vi "Begin.vi"(8 "error in":errorcluster) -> (0 "error out":errorcluster)   [LabVIEW 2019]
doc: "Called before other user functions, this VI can be used to open I/O refnums, load in file data, and do general program initialization. Notice that the <B>error out</B> terminal is simply used for data flow. Wiring it to other structures or subVIs ensures that this VI runs first."
uses:
  Robot Global Data.vi
  <vilib>/Rock Robotics/WPI/DriverStation/WPI_DriverStationRobotMode2.ctl
  <vilib>/Rock Robotics/WPI/Joystick/WPI_JoystickDeviceEnum.ctl
  <vilib>/Rock Robotics/Network Tables/NT Write String Array.vi
  <vilib>/Rock Robotics/WPI/RobotDrive/WPI_RobotDriveOpen2MotorWithExistingMotors.vi
  <vilib>/Rock Robotics/WPI/MotorControl/WPI_MotorControlOpen SPARK.vi
  <vilib>/Rock Robotics/SystemInterfaces/DIO/FPGA_DIOPWMChannel.ctl
  <vilib>/Rock Robotics/WPI/SafetyOutput/WPI_SafetyOutputConfigMenu.ctl
  <vilib>/Rock Robotics/Network Tables/NT Write Numeric Array.vi
  <vilib>/Rock Robotics/Network Tables/NT Write Boolean Array.vi
  <vilib>/Rock Robotics/WPI/Solenoid/WPI_SolenoidOpenSingle.vi
  <vilib>/Rock Robotics/WPI/Solenoid/WPI_SolenoidSetEnum.vi
  <vilib>/Rock Robotics/WPI/Solenoid/WPI_SolenoidChannel.ctl
  <vilib>/Rock Robotics/WPI/Solenoid/WPI_SolenoidValue.ctl
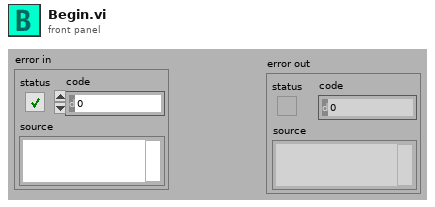
[diagram p1: front panel]
types:
  T1 = typedef "WPI_JoystickDeviceEnum.ctl" = enum16{"USB 0", "USB 1", "USB 2", "USB 3", "USB 4", "USB 5"}
  T2 = typedef "WPI_DriverStationRobotMode2.ctl" = enum16{"Autonomous Disabled", "Autonomous Enabled", "Teleop Disabled", "Teleop Enabled", "Disconnected", "Finish", "Test Disabled", "Test Enabled", "Emergency Stopped"}
  T3 = typedef "WPI_JoystickDevRef.ctl" = cluster{"Device":T1}
  T4 = typedef "WPI_MotorControlDeviceRef.ctl" = cluster{"DeviceStatus":errorcluster, "Type":T5, "PWM":cluster{"PWM Channel":T6, "DeadBand":T7}, "CAN":cluster{"Device Number":u8, "SetOutput VI Ref":variant, "GetOutput VI Ref":variant, "Enable VI Ref":variant, "Disable VI Ref":variant, "Data":variant}, "Invert":bool, "DIO PWM":cluster{"PWM \"Enable\" Channel":T6, "DIOChannel":T8, "PWM Rate":dbl}}
  T5 = typedef "WPI_MotorControlType.ctl" = enum16{"PWM", "CAN", "DIO PWM"}
  T6 = typedef "FPGA_DIOPWMChannel.ctl" = enum8{"PWM 0", "PWM 1", "PWM 2", "PWM 3", "PWM 4", "PWM 5", "PWM 6", "PWM 7", "PWM 8", "PWM 9", "PWM MXP 0", "PWM MXP 1", "PWM MXP 2", "PWM MXP 3", "PWM MXP 4", "PWM MXP 5", "PWM MXP 6", "PWM MXP 7", "PWM MXP 8", "PWM MXP 9", "Invalid"}
  T7 = typedef "WPI_PWMDeadband.ctl" = cluster{"Name":string, "maxPositivePwm":i32, "minPositivePwm":i32, "centerPwm":i32, "maxNegativePwm":i32, "minNegativePwm":i32, "angularRange":u16}
  T8 = typedef "FPGA_DIOChannel.ctl" = enum8{"DIO 0", "DIO 1", "DIO 2", "DIO 3", "DIO 4", "DIO 5", "DIO 6", "DIO 7", "DIO 8", "DIO 9", "DIO MXP 0", "DIO MXP 1", "DIO MXP 2", "DIO MXP 3", "DIO MXP 4", "DIO MXP 5", "DIO MXP 6", "DIO MXP 7", "DIO MXP 8", "DIO MXP 9", "DIO MXP 10", "DIO MXP 11", "DIO MXP 12", "DIO MXP 13", "DIO MXP 14", "DIO MXP 15", "SPI Port CS1", "SPI Port CS2", "SPI Port CS3", "SPI Port MISO", "SPI Port MOSI", "Invalid"}
  T9 = typedef "WPI_SafetyOutputConfigMenu.ctl" = enum16{"Enable", "Disable"}
  T10 = typedef "WPI_RobotDriveDevRef.ctl" = cluster{"DevStatus":errorcluster, "Motors[]":T4[], "Square Inputs":bool, "Max Output":dbl}
  T11 = typedef "WPI_SolenoidValue.ctl" = enum16{"Off", "On", "Forward", "Reverse"}
  T12 = typedef "WPI_SolenoidChannel.ctl" = enum8{"Solenoid 0", "Solenoid 1", "Solenoid 2", "Solenoid 3", "Solenoid 4", "Solenoid 5", "Solenoid 6", "Solenoid 7", "Invalid"}
  T13 = typedef "WPI_SolenoidDevRef.ctl" = cluster{"DevStatus":errorcluster, "Pneumatics Control Module":u8, "Forward Solenoid Channel":T12, "Reverse Solenoid Channel":T12}
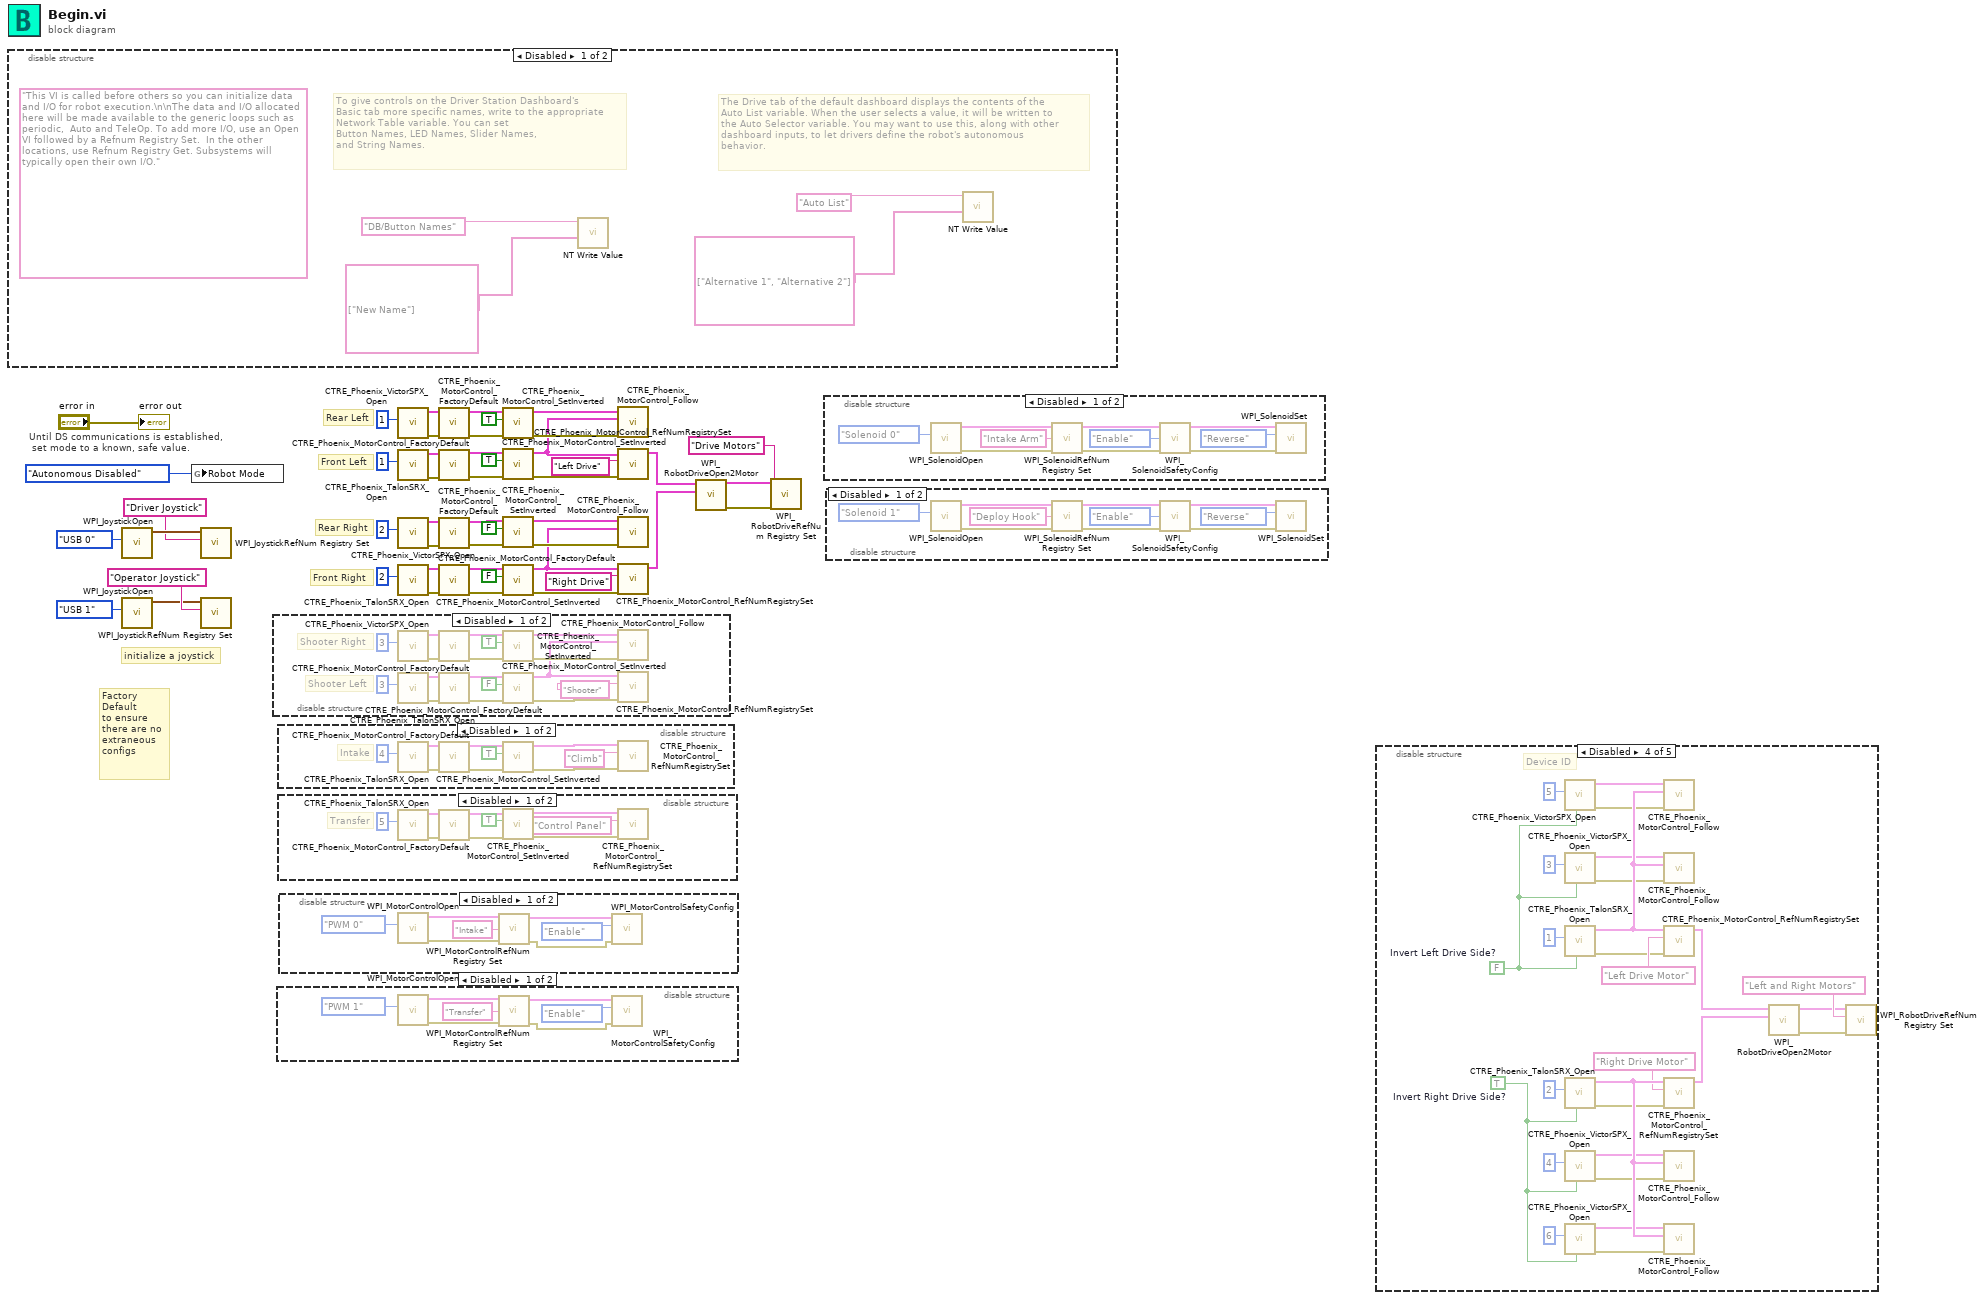
[diagram p0: block diagram]
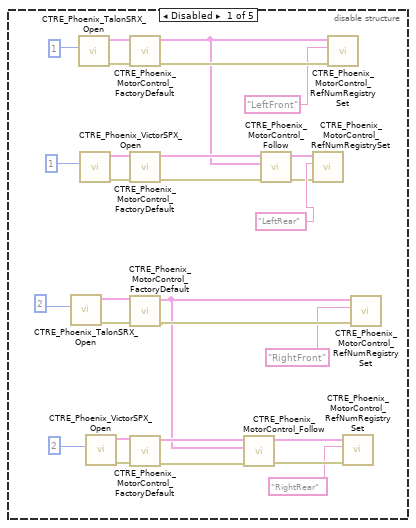
[diagram p9: hidden frame]
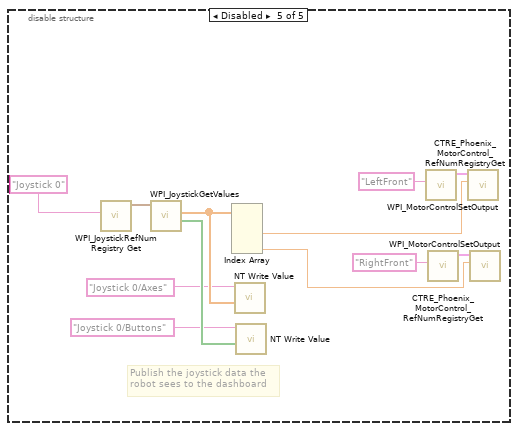
[diagram p12: hidden frame]
diagram:
  # "Factory \nDefault \nto ensure \nthere are no \nextraneous \nconfigs"
  # "Front Right"
  # "Front Left"
  # "Rear Right"
  # "Rear Left"
  # "initialize a joystick"
  # "Until DS communications is established,\n set mode to a known, safe value."
  n1 = disable-structure shown="Disabled" {
    frame Disabled {
      (unwired) "This VI is called before others so you can initialize data and I/O for robot execution.\n\nThe data and I/O allocated here will be made available to the generic loops such as periodic,  Auto and TeleOp. To add more I/O, use an Open VI followed by a Refnum Registry Set.  In the other locations, use Refnum Registry Get. Subsystems will typically open their own I/O."
      # "The Drive tab of the default dashboard displays the contents of the\nAuto List variable. When the user selects a value, it will be written to\nthe Auto Selector variable. You may want to use this, along with other\ndashboard inputs, to let drivers define the robot's autonomous\nbehavior."
      # "To give controls on the Driver Station Dashboard's\nBasic tab more specific names, write to the appropriate\nNetwork Table variable. You can set\nButton Names, LED Names, Slider Names,\nand String Names."
      n2 = call-poly <vilib>:"NT Write Value.vi"("String Array"=string[] ["New Name"], "Name"="DB/Button Names") -> ()  [unwired: 9 in, 1 out]
      n3 = call-poly <vilib>:"NT Write Value.vi"("String Array"=string[] ["Alternative 1", "Alternative 2"], "Name"="Auto List") -> ()  [unwired: 9 in, 1 out]
    }
    frame Enabled {
    }
  }
  n4 = call <vilib>:"WPI_JoystickOpen.vi"("JoystickDevice"=WPI_JoystickDeviceEnum."USB 0") -> ("JoystickDevRef"=w30:T3)  [unwired: 10 in]
  n5 = call <vilib>:"WPI_JoystickOpen.vi"("JoystickDevice"=WPI_JoystickDeviceEnum."USB 1") -> ("JoystickDevRef"=w45:T3)  [unwired: 10 in]
  n6 = global write "Robot Global Data.vi" "Robot Mode"(WPI_DriverStationRobotMode2."Autonomous Disabled" ("Robot Mode")) -> ()
  n7 = call <vilib>:"WPI_JoystickRefNum Registry Set.vi"("refnum name"="Driver Joystick", "JoystickDevRef"=w30) -> ()  [unwired: 8 in, 2 out]
  n8 = call <vilib>:"WPI_JoystickRefNum Registry Set.vi"("refnum name"="Operator Joystick", "JoystickDevRef"=w45) -> ()  [unwired: 8 in, 2 out]
  n9 = disable-structure shown="Disabled" {
    frame Disabled {
      # "Shooter Left"
      # "Shooter Right"
      n10 = call <vilib>:"CTRE_Phoenix_VictorSPX_Open.vi"("Device Number"=u8 3) -> ("error out"=w65:errorcluster, "CAN Talon SRX Ref"=w64:T4)  [unwired: 9 in]
      n11 = call <vilib>:"CTRE_Phoenix_TalonSRX_Open.vi"("Device Number"=u8 3) -> ("error out"=w63:errorcluster, "CAN Talon SRX Ref"=w62:T4)  [unwired: 9 in]
      n12 = call <vilib>:"CTRE_Phoenix_MotorControl_FactoryDefault.vi"("error in"=w65, "PhoenixMotorControlDevRef"=w64) -> ("error out"=w59:errorcluster, "PhoenixMotorControlDevRef"=w60:T4)  [unwired: 8 in]
      n13 = call <vilib>:"CTRE_Phoenix_MotorControl_FactoryDefault.vi"("error in"=w63, "PhoenixMotorControlDevRef"=w62) -> ("error out"=w54:errorcluster, "PhoenixMotorControlDevRef"=w55:T4)  [unwired: 8 in]
      n14 = call <vilib>:"CTRE_Phoenix_MotorControl_SetInverted.vi"("error in (no error)"=w59, "Invert?"=TRUE, "PhoenixMotorControlDevRef"=w60) -> ("error out"=w58:errorcluster, "PhoenixMotorControlDevRef"=w57:T4)  [unwired: 7 in]
      n15 = call <vilib>:"CTRE_Phoenix_MotorControl_SetInverted.vi"("error in (no error)"=w54, "Invert?"=FALSE, "PhoenixMotorControlDevRef"=w55) -> ("error out"=w53:errorcluster, "PhoenixMotorControlDevRef"=w52:T4)  [unwired: 7 in]
      n16 = call <vilib>:"CTRE_Phoenix_MotorControl_Follow.vi"("error in (no error)"=w58, "Master Controller to Follow"=w52, "PhoenixMotorControlDevRef"=w57) -> ()  [unwired: 7 in, 2 out]
      n17 = call <vilib>:"CTRE_Phoenix_MotorControl_RefNumRegistrySet.vi"("error in (no error)"=w53, "refnum name"="Shooter", "PhoenixMotorControlDevRef"=w52) -> ()  [unwired: 7 in, 2 out]
    }
    frame Enabled {
    }
  }
  n18 = disable-structure shown="Disabled" {
    frame Disabled {
      n19 = call-poly <vilib>:"WPI_MotorControlOpen.vi"("PWM Channel"=FPGA_DIOPWMChannel."PWM 1") -> ("error out"=w74:errorcluster, "MotorControlDeviceRef"=w70:T4)  [unwired: 9 in]
      n20 = call <vilib>:"WPI_MotorControlRefNum Registry Set.vi"("error in (no error)"=w74, "refnum name"="Transfer", "MotorControlDevRef"=w70) -> ("error out"=w75:errorcluster, "MotorControlDevRef"=w71:T4)  [unwired: 7 in]
      n21 = call <vilib>:"WPI_MotorControlSafetyConfig.vi"("error in (no error)"=w75, "mode"=WPI_SafetyOutputConfigMenu."Enable", "MotorControlDevRef"=w71) -> ()  [unwired: 7 in, 2 out]
    }
    frame Enabled {
    }
  }
  n22 = disable-structure shown="Disabled" {
    frame Disabled {
      # "Intake"
      n23 = call <vilib>:"CTRE_Phoenix_TalonSRX_Open.vi"("Device Number"=u8 4) -> ("error out"=w82:errorcluster, "CAN Talon SRX Ref"=w81:T4)  [unwired: 9 in]
      n24 = call <vilib>:"CTRE_Phoenix_MotorControl_FactoryDefault.vi"("error in"=w82, "PhoenixMotorControlDevRef"=w81) -> ("error out"=w78:errorcluster, "PhoenixMotorControlDevRef"=w79:T4)  [unwired: 8 in]
      n25 = call <vilib>:"CTRE_Phoenix_MotorControl_SetInverted.vi"("error in (no error)"=w78, "Invert?"=TRUE, "PhoenixMotorControlDevRef"=w79) -> ("error out"=w77:errorcluster, "PhoenixMotorControlDevRef"=w76:T4)  [unwired: 7 in]
      n26 = call <vilib>:"CTRE_Phoenix_MotorControl_RefNumRegistrySet.vi"("error in (no error)"=w77, "refnum name"="Climb", "PhoenixMotorControlDevRef"=w76) -> ()  [unwired: 7 in, 2 out]
    }
    frame Enabled {
    }
  }
  n27 = disable-structure shown="Disabled" {
    frame Disabled {
      # "Transfer"
      n28 = call <vilib>:"CTRE_Phoenix_TalonSRX_Open.vi"("Device Number"=u8 5) -> ("error out"=w91:errorcluster, "CAN Talon SRX Ref"=w90:T4)  [unwired: 9 in]
      n29 = call <vilib>:"CTRE_Phoenix_MotorControl_FactoryDefault.vi"("error in"=w91, "PhoenixMotorControlDevRef"=w90) -> ("error out"=w87:errorcluster, "PhoenixMotorControlDevRef"=w88:T4)  [unwired: 8 in]
      n30 = call <vilib>:"CTRE_Phoenix_MotorControl_SetInverted.vi"("error in (no error)"=w87, "Invert?"=TRUE, "PhoenixMotorControlDevRef"=w88) -> ("error out"=w86:errorcluster, "PhoenixMotorControlDevRef"=w85:T4)  [unwired: 7 in]
      n31 = call <vilib>:"CTRE_Phoenix_MotorControl_RefNumRegistrySet.vi"("error in (no error)"=w86, "refnum name"="Control Panel", "PhoenixMotorControlDevRef"=w85) -> ()  [unwired: 7 in, 2 out]
    }
    frame Enabled {
    }
  }
  n32 = disable-structure shown="Disabled" {
    frame Disabled {
      n33 = call-poly <vilib>:"WPI_MotorControlOpen.vi"("PWM Channel"=FPGA_DIOPWMChannel."PWM 0") -> ("error out"=w95:errorcluster, "MotorControlDeviceRef"=w99:T4)  [unwired: 9 in]
      n34 = call <vilib>:"WPI_MotorControlRefNum Registry Set.vi"("error in (no error)"=w95, "refnum name"="Intake", "MotorControlDevRef"=w99) -> ("error out"=w94:errorcluster, "MotorControlDevRef"=w98:T4)  [unwired: 7 in]
      n35 = call <vilib>:"WPI_MotorControlSafetyConfig.vi"("error in (no error)"=w94, "mode"=WPI_SafetyOutputConfigMenu."Enable", "MotorControlDevRef"=w98) -> ()  [unwired: 7 in, 2 out]
    }
    frame Enabled {
    }
  }
  n36 = call <vilib>:"CTRE_Phoenix_VictorSPX_Open.vi"("Device Number"=u8 1) -> ("error out"=w28:errorcluster, "CAN Talon SRX Ref"=w27:T4)  [unwired: 9 in]
  n37 = call <vilib>:"CTRE_Phoenix_TalonSRX_Open.vi"("Device Number"=u8 1) -> ("error out"=w25:errorcluster, "CAN Talon SRX Ref"=w26:T4)  [unwired: 9 in]
  n38 = call <vilib>:"CTRE_Phoenix_VictorSPX_Open.vi"("Device Number"=u8 2) -> ("error out"=w24:errorcluster, "CAN Talon SRX Ref"=w23:T4)  [unwired: 9 in]
  n39 = call <vilib>:"CTRE_Phoenix_TalonSRX_Open.vi"("Device Number"=u8 2) -> ("error out"=w22:errorcluster, "CAN Talon SRX Ref"=w21:T4)  [unwired: 9 in]
  n40 = call <vilib>:"CTRE_Phoenix_MotorControl_FactoryDefault.vi"("error in"=w28, "PhoenixMotorControlDevRef"=w27) -> ("error out"=w19:errorcluster, "PhoenixMotorControlDevRef"=w18:T4)  [unwired: 8 in]
  n41 = call <vilib>:"CTRE_Phoenix_MotorControl_FactoryDefault.vi"("error in"=w25, "PhoenixMotorControlDevRef"=w26) -> ("error out"=w13:errorcluster, "PhoenixMotorControlDevRef"=w14:T4)  [unwired: 8 in]
  n42 = call <vilib>:"CTRE_Phoenix_MotorControl_FactoryDefault.vi"("error in"=w24, "PhoenixMotorControlDevRef"=w23) -> ("error out"=w9:errorcluster, "PhoenixMotorControlDevRef"=w8:T4)  [unwired: 8 in]
  n43 = call <vilib>:"CTRE_Phoenix_MotorControl_FactoryDefault.vi"("error in"=w22, "PhoenixMotorControlDevRef"=w21) -> ("error out"=w4:errorcluster, "PhoenixMotorControlDevRef"=w3:T4)  [unwired: 8 in]
  n44 = call <vilib>:"CTRE_Phoenix_MotorControl_SetInverted.vi"("error in (no error)"=w19, "Invert?"=TRUE, "PhoenixMotorControlDevRef"=w18) -> ("error out"=w16:errorcluster, "PhoenixMotorControlDevRef"=w17:T4)  [unwired: 7 in]
  n45 = call <vilib>:"CTRE_Phoenix_MotorControl_SetInverted.vi"("error in (no error)"=w13, "Invert?"=TRUE, "PhoenixMotorControlDevRef"=w14) -> ("error out"=w12:errorcluster, "PhoenixMotorControlDevRef"=w11:T4)  [unwired: 7 in]
  n46 = call <vilib>:"CTRE_Phoenix_MotorControl_SetInverted.vi"("error in (no error)"=w9, "Invert?"=FALSE, "PhoenixMotorControlDevRef"=w8) -> ("error out"=w6:errorcluster, "PhoenixMotorControlDevRef"=w7:T4)  [unwired: 7 in]
  n47 = call <vilib>:"CTRE_Phoenix_MotorControl_SetInverted.vi"("error in (no error)"=w4, "Invert?"=FALSE, "PhoenixMotorControlDevRef"=w3) -> ("error out"=w1:errorcluster, "PhoenixMotorControlDevRef"=w2:T4)  [unwired: 7 in]
  n48 = call <vilib>:"CTRE_Phoenix_MotorControl_Follow.vi"("error in (no error)"=w16, "Master Controller to Follow"=w11, "PhoenixMotorControlDevRef"=w17) -> ()  [unwired: 7 in, 2 out]
  n49 = call <vilib>:"CTRE_Phoenix_MotorControl_RefNumRegistrySet.vi"("error in (no error)"=w12, "refnum name"="Left Drive", "PhoenixMotorControlDevRef"=w11) -> ("PhoenixMotorControlDevRef"=w38:T4)  [unwired: 7 in, 1 out]
  n50 = call <vilib>:"CTRE_Phoenix_MotorControl_Follow.vi"("error in (no error)"=w6, "Master Controller to Follow"=w2, "PhoenixMotorControlDevRef"=w7) -> ()  [unwired: 7 in, 2 out]
  n51 = call <vilib>:"CTRE_Phoenix_MotorControl_RefNumRegistrySet.vi"("error in (no error)"=w1, "refnum name"="Right Drive", "PhoenixMotorControlDevRef"=w2) -> ("PhoenixMotorControlDevRef"=w37:T4)  [unwired: 7 in, 1 out]
  n52 = call-poly <vilib>:"WPI_RobotDriveOpen2Motor.vi"("Right Motor Dev Ref"=w37, "Left Motor Dev Ref"=w38) -> ("error out"=w33:errorcluster, "RobotDriveDevRef"=w34:T10)  [unwired: 8 in]
  n53 = call <vilib>:"WPI_RobotDriveRefNum Registry Set.vi"("error in (no error)"=w33, "refnum name"="Drive Motors", "RobotDriveDevRef"=w34) -> ()  [unwired: 7 in, 2 out]
  n54 = disable-structure shown="Disabled" {
    frame Disabled {
      n55 = call-poly <vilib>:"WPI_SolenoidOpen.vi"("Solenoid Channel"=WPI_SolenoidChannel."Solenoid 0") -> ("error out"=w107:errorcluster, "SolenoidDevRef"=w110:T13)  [unwired: 9 in]
      n56 = call <vilib>:"WPI_SolenoidRefNum Registry Set.vi"("error in (no error)"=w107, "refnum name"="Intake Arm", "SolenoidDevRef"=w110) -> ("error out"=w106:errorcluster, "SolenoidDevRef"=w109:T13)  [unwired: 7 in]
      n57 = call <vilib>:"WPI_SolenoidSafetyConfig.vi"("error in (no error)"=w106, "mode"=WPI_SafetyOutputConfigMenu."Enable", "SolenoidDevRef"=w109) -> ("error out"=w105:errorcluster, "SolenoidDevRef"=w108:T13)  [unwired: 7 in]
      n58 = call-poly <vilib>:"WPI_SolenoidSet.vi"("error in (no error)"=w105, "Value"=WPI_SolenoidValue."Reverse", "SolenoidDevRef"=w108) -> ()  [unwired: 7 in, 2 out]
    }
    frame Enabled {
    }
  }
  n59 = disable-structure shown="Disabled" {
    frame Disabled {
      n60 = call-poly <vilib>:"WPI_SolenoidOpen.vi"("Solenoid Channel"=WPI_SolenoidChannel."Solenoid 1") -> ("error out"=w114:errorcluster, "SolenoidDevRef"=w111:T13)  [unwired: 9 in]
      n61 = call <vilib>:"WPI_SolenoidRefNum Registry Set.vi"("error in (no error)"=w114, "refnum name"="Deploy Hook", "SolenoidDevRef"=w111) -> ("error out"=w115:errorcluster, "SolenoidDevRef"=w112:T13)  [unwired: 7 in]
      n62 = call <vilib>:"WPI_SolenoidSafetyConfig.vi"("error in (no error)"=w115, "mode"=WPI_SafetyOutputConfigMenu."Enable", "SolenoidDevRef"=w112) -> ("error out"=w116:errorcluster, "SolenoidDevRef"=w113:T13)  [unwired: 7 in]
      n63 = call-poly <vilib>:"WPI_SolenoidSet.vi"("error in (no error)"=w116, "Value"=WPI_SolenoidValue."Reverse", "SolenoidDevRef"=w113) -> ()  [unwired: 7 in, 2 out]
    }
    frame Enabled {
    }
  }
  n64 = disable-structure shown="Disabled" {
    frame Disabled {
      n65 = call <vilib>:"CTRE_Phoenix_TalonSRX_Open.vi"("Device Number"=u8 2) -> ("error out"=w145:errorcluster, "CAN Talon SRX Ref"=w135:T4)  [unwired: 9 in]
      n66 = call <vilib>:"CTRE_Phoenix_TalonSRX_Open.vi"("Device Number"=u8 1) -> ("error out"=w143:errorcluster, "CAN Talon SRX Ref"=w133:T4)  [unwired: 9 in]
      n67 = call <vilib>:"CTRE_Phoenix_VictorSPX_Open.vi"("Device Number"=u8 1) -> ("error out"=w141:errorcluster, "CAN Talon SRX Ref"=w139:T4)  [unwired: 9 in]
      n68 = call <vilib>:"CTRE_Phoenix_VictorSPX_Open.vi"("Device Number"=u8 2) -> ("error out"=w147:errorcluster, "CAN Talon SRX Ref"=w137:T4)  [unwired: 9 in]
      n69 = call <vilib>:"CTRE_Phoenix_MotorControl_FactoryDefault.vi"("error in"=w143, "PhoenixMotorControlDevRef"=w133) -> ("error out"=w144:errorcluster, "PhoenixMotorControlDevRef"=w134:T4)  [unwired: 8 in]
      n70 = call <vilib>:"CTRE_Phoenix_MotorControl_FactoryDefault.vi"("error in"=w141, "PhoenixMotorControlDevRef"=w139) -> ("error out"=w142:errorcluster, "PhoenixMotorControlDevRef"=w140:T4)  [unwired: 8 in]
      n71 = call <vilib>:"CTRE_Phoenix_MotorControl_FactoryDefault.vi"("error in"=w145, "PhoenixMotorControlDevRef"=w135) -> ("error out"=w146:errorcluster, "PhoenixMotorControlDevRef"=w136:T4)  [unwired: 8 in]
      n72 = call <vilib>:"CTRE_Phoenix_MotorControl_FactoryDefault.vi"("error in"=w147, "PhoenixMotorControlDevRef"=w137) -> ("error out"=w148:errorcluster, "PhoenixMotorControlDevRef"=w138:T4)  [unwired: 8 in]
      n73 = call <vilib>:"CTRE_Phoenix_MotorControl_Follow.vi"("error in (no error)"=w148, "Master Controller to Follow"=w136, "PhoenixMotorControlDevRef"=w138) -> ("error out"=w131:errorcluster, "PhoenixMotorControlDevRef"=w132:T4)  [unwired: 7 in]
      n74 = call <vilib>:"CTRE_Phoenix_MotorControl_Follow.vi"("error in (no error)"=w142, "Master Controller to Follow"=w134, "PhoenixMotorControlDevRef"=w140) -> ("error out"=w123:errorcluster, "PhoenixMotorControlDevRef"=w124:T4)  [unwired: 7 in]
      n75 = call <vilib>:"CTRE_Phoenix_MotorControl_RefNumRegistrySet.vi"("error in (no error)"=w123, "refnum name"="LeftRear", "PhoenixMotorControlDevRef"=w124) -> ()  [unwired: 7 in, 2 out]
      n76 = call <vilib>:"CTRE_Phoenix_MotorControl_RefNumRegistrySet.vi"("error in (no error)"=w144, "refnum name"="LeftFront", "PhoenixMotorControlDevRef"=w134) -> ()  [unwired: 7 in, 2 out]
      n77 = call <vilib>:"CTRE_Phoenix_MotorControl_RefNumRegistrySet.vi"("error in (no error)"=w131, "refnum name"="RightRear", "PhoenixMotorControlDevRef"=w132) -> ()  [unwired: 7 in, 2 out]
      n78 = call <vilib>:"CTRE_Phoenix_MotorControl_RefNumRegistrySet.vi"("error in (no error)"=w146, "refnum name"="RightFront", "PhoenixMotorControlDevRef"=w136) -> ()  [unwired: 7 in, 2 out]
    }
    frame Enabled {
    }
    frame Disabled {
    }
    frame Disabled {
      w175 = FALSE  # Invert Left Drive Side?
      w174 = TRUE  # Invert Right Drive Side?
      # "Device ID"
      n79 = call <vilib>:"CTRE_Phoenix_VictorSPX_Open.vi"("Invert"=w175, "Device Number"=u8 5) -> ("error out"=w165:errorcluster, "CAN Talon SRX Ref"=w166:T4)  [unwired: 8 in]
      n80 = call <vilib>:"CTRE_Phoenix_VictorSPX_Open.vi"("Invert"=w175, "Device Number"=u8 3) -> ("error out"=w164:errorcluster, "CAN Talon SRX Ref"=w167:T4)  [unwired: 8 in]
      n81 = call <vilib>:"CTRE_Phoenix_TalonSRX_Open.vi"("Invert"=w175, "Device Number"=u8 1) -> ("error out"=w155:errorcluster, "CAN Talon SRX Ref"=w168:T4)  [unwired: 8 in]
      n82 = call <vilib>:"CTRE_Phoenix_TalonSRX_Open.vi"("Invert"=w174, "Device Number"=u8 2) -> ("error out"=w156:errorcluster, "CAN Talon SRX Ref"=w163:T4)  [unwired: 8 in]
      n83 = call <vilib>:"CTRE_Phoenix_VictorSPX_Open.vi"("Invert"=w174, "Device Number"=u8 4) -> ("error out"=w159:errorcluster, "CAN Talon SRX Ref"=w160:T4)  [unwired: 8 in]
      n84 = call <vilib>:"CTRE_Phoenix_VictorSPX_Open.vi"("Invert"=w174, "Device Number"=u8 6) -> ("error out"=w162:errorcluster, "CAN Talon SRX Ref"=w161:T4)  [unwired: 8 in]
      n85 = call <vilib>:"CTRE_Phoenix_MotorControl_Follow.vi"("error in (no error)"=w165, "Master Controller to Follow"=w168, "PhoenixMotorControlDevRef"=w166) -> ()  [unwired: 7 in, 2 out]
      n86 = call <vilib>:"CTRE_Phoenix_MotorControl_Follow.vi"("error in (no error)"=w164, "Master Controller to Follow"=w168, "PhoenixMotorControlDevRef"=w167) -> ()  [unwired: 7 in, 2 out]
      n87 = call <vilib>:"CTRE_Phoenix_MotorControl_RefNumRegistrySet.vi"("error in (no error)"=w155, "refnum name"="Left Drive Motor", "PhoenixMotorControlDevRef"=w168) -> ("PhoenixMotorControlDevRef"=w169:T4)  [unwired: 7 in, 1 out]
      n88 = call <vilib>:"CTRE_Phoenix_MotorControl_RefNumRegistrySet.vi"("error in (no error)"=w156, "refnum name"="Right Drive Motor", "PhoenixMotorControlDevRef"=w163) -> ("PhoenixMotorControlDevRef"=w170:T4)  [unwired: 7 in, 1 out]
      n89 = call <vilib>:"CTRE_Phoenix_MotorControl_Follow.vi"("error in (no error)"=w159, "Master Controller to Follow"=w163, "PhoenixMotorControlDevRef"=w160) -> ()  [unwired: 7 in, 2 out]
      n90 = call <vilib>:"CTRE_Phoenix_MotorControl_Follow.vi"("error in (no error)"=w162, "Master Controller to Follow"=w163, "PhoenixMotorControlDevRef"=w161) -> ()  [unwired: 7 in, 2 out]
      n91 = call-poly <vilib>:"WPI_RobotDriveOpen2Motor.vi"("Right Motor Dev Ref"=w170, "Left Motor Dev Ref"=w169) -> ("error out"=w171:errorcluster, "RobotDriveDevRef"=w172:T10)  [unwired: 8 in]
      n92 = call <vilib>:"WPI_RobotDriveRefNum Registry Set.vi"("error in (no error)"=w171, "refnum name"="Left and Right Motors", "RobotDriveDevRef"=w172) -> ()  [unwired: 7 in, 2 out]
    }
    frame Disabled {
      # "Publish the joystick data the\nrobot sees to the dashboard"
      n93 = call <vilib>:"WPI_JoystickRefNum Registry Get.vi"("refnum name"="Joystick 0") -> ("JoystickDevRef"=w177:T3)  [unwired: 1 in, 9 out]
      n94 = call <vilib>:"WPI_JoystickGetValues.vi"("JoystickDevRef"=w177) -> ("Buttons"=w181:bool[], "Axes"=w180:dbl[])  [unwired: 6 in, 3 out]
      n95 = Index Array(array=w180) -> (element #2=w184:dbl, element #4=w187:dbl)  [unwired: 4 in, 2 out]
      n96 = call-poly <vilib>:"NT Write Value.vi"("Numeric Array"=w180, "Name"="Joystick 0/Axes") -> ()  [unwired: 9 in, 1 out]
      n97 = call-poly <vilib>:"NT Write Value.vi"("Boolean Array"=w181, "Name"="Joystick 0/Buttons") -> ()  [unwired: 9 in, 1 out]
      n98 = call <vilib>:"CTRE_Phoenix_MotorControl_RefNumRegistryGet.vi"("refnum name"="LeftFront") -> ("PhoenixMotorControlDevRef"=w183:T4)  [unwired: 9 in, 1 out]
      n99 = call <vilib>:"CTRE_Phoenix_MotorControl_RefNumRegistryGet.vi"("refnum name"="RightFront") -> ("PhoenixMotorControlDevRef"=w186:T4)  [unwired: 9 in, 1 out]
      n100 = call <vilib>:"WPI_MotorControlSetOutput.vi"("Output"=w184, "MotorControlDevRef"=w183) -> ()  [unwired: 7 in, 3 out]
      n101 = call <vilib>:"WPI_MotorControlSetOutput.vi"("Output"=w187, "MotorControlDevRef"=w186) -> ()  [unwired: 7 in, 3 out]
    }
  }
  "error out" <- "error in"
